vi "NF WF1973_74 CHAN Rat.vi"(0 "VISAsession":refnum<visa-resource-name>, 1 "Set Ch1 Ratio(Input)":u16(ring) items=["Input", "Minimum", "Maximum"], 2 "Set Ch2 Ratio(Input)":u16(ring) items=["Input", "Minimum", "Maximum"], 5 "Ch1(1)":i32=1 min=1 max=9999999 step=1, 7 "Ch2(1)":i32=1 min=1 max=9999999 step=1, 11 "error in (no error)":errorcluster caption="Error IN", 12 "Read(F)":bool) -> (4 "CopyVISAsession":refnum<visa-resource-name>, 6 "Query Ratio":string, 15 "error out":errorcluster caption="Error OUT")   [LabVIEW 2010]
panel:
  # "Choose\nInput"
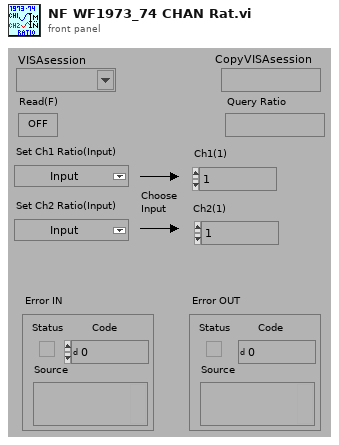
[diagram p1: front panel]
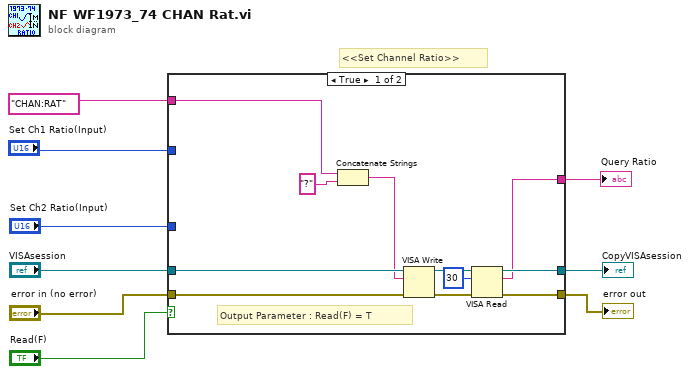
[diagram p0: block diagram]
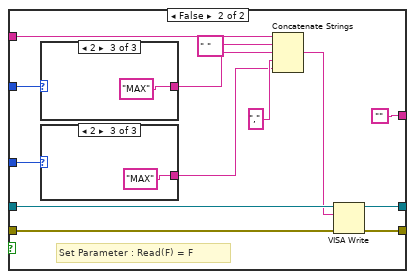
[diagram p2: hidden frame]
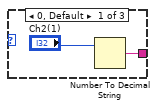
[diagram p3: hidden frame]
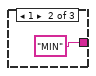
[diagram p4: hidden frame]
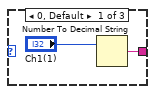
[diagram p5: hidden frame]
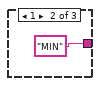
[diagram p6: hidden frame]
diagram:
  # "<<Set Channel Ratio>>"
  n1 = case shown="TRUE" "Read(F)" {
    tunnel: "VISAsession" -> [w20 w33]
    tunnel: [w17 w30] -> w8
    tunnel: [w16 w31] -> w7
    tunnel: "error in (no error)" -> [w15 w32]
    tunnel: "CHAN:RAT" ("文字列") -> [w13 w26]
    tunnel: [w11 ""] -> w3
    tunnel: "Set Ch1 Ratio(Input)" -> [_ w22]
    tunnel: "Set Ch2 Ratio(Input)" -> [_ w21]
    frame True {
      # "Output Parameter : Read(F) = T"
      n2 = Concatenate Strings(w13, "?" ("形式文字列")) -> (w12:string)
      n3 = VISA Write(VISA resource name=w20, write buffer=w12, error in (no error)=w15) -> (VISA resource name out=w18:refnum<visa-resource-name>, error out=w19:errorcluster)  [unwired: 1 out]
      n4 = VISA Read(VISA resource name=w18, byte count=u32 30 ("バイトカウント（0）"), error in (no error)=w19) -> (VISA resource name out=w17:refnum<visa-resource-name>, read buffer=w11:string, error out=w16:errorcluster)  [unwired: 1 out]
    }
    frame False {
      # "Set Parameter : Read(F) = F"
      n5 = case shown="2" w22 {
        tunnel: [w39 "MIN" ("文字列") "MAX" ("文字列")] -> w24
        frame 0, Default {
          n6 = Number To Decimal String(number="Ch1(1)") -> (decimal integer string=w39:string)  [unwired: 1 in]
        }
        frame 1 {
        }
        frame 2 {
        }
      }
      n7 = case shown="2" w21 {
        tunnel: [w35 "MIN" ("文字列") "MAX" ("文字列")] -> w23
        frame 0, Default {
          n8 = Number To Decimal String(number="Ch2(1)") -> (decimal integer string=w35:string)  [unwired: 1 in]
        }
        frame 1 {
        }
        frame 2 {
        }
      }
      n9 = Concatenate Strings(w26, " ", w24, "," ("文字列"), w23) -> (w28:string)
      n10 = VISA Write(VISA resource name=w33, write buffer=w28, error in (no error)=w32) -> (VISA resource name out=w30:refnum<visa-resource-name>, error out=w31:errorcluster)  [unwired: 1 out]
    }
  }
  "error out" <- w7
  "CopyVISAsession" <- w8
  "Query Ratio" <- w3
